vi "GetFuncGenMaxAmplitude.vi"(8 "error in (no error)":errorcluster, 11 "dAmplitude":dbl) -> (0 "error out":errorcluster, 2 "function return":i16, 3 "dAmplitude out":dbl)   [LabVIEW 2013, in "HS3OverallRoutines.lvlib"]
doc: "short int GetFuncGenMaxAmplitude ( double *dAmplitude );"
uses:
  HS3OverallRoutines.lvlib
  hs3.dll
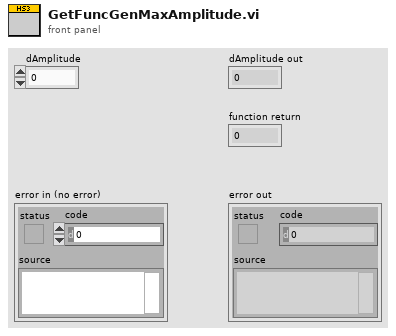
[diagram p1: front panel]
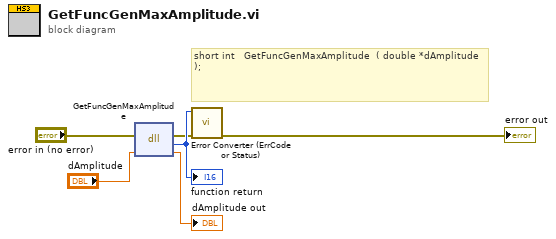
[diagram p0: block diagram]
diagram:
  # "short int \t\tGetFuncGenMaxAmplitude\t\t( double *dAmplitude );"
  n1 = dll-call lib="C:/Documents and Settings/admin/Pulpit/HS3 LabViewLib/HS3_WRAPPER/OverallRoutines/hs3.*" fn="GetFuncGenMaxAmplitude"(error in="error in (no error)", "dAmplitude"="dAmplitude") -> (error out=w2:errorcluster, w6:i16, "dAmplitude"=→"dAmplitude out":dbl)  [unwired: 2 in, 1 out]
  "function return" <- w6
  n2 = call "Error Converter (ErrCode or Status).vi"("error in (no error)"=w2, "error code"=w6) -> ("error out"=→"error out":errorcluster)  [unwired: 9 in]
